vi "PIDController_AdvCalculate_FF_Sp_Pv_Per.vi"(6 "Period":dbl, 7 "Auto":bool=TRUE, 8 "FF":dbl, 9 "SP":dbl, 10 "PV":dbl, 11 "in PID_CONTROLLER":T1={"Kp"=0.0, "Ki"=0.0, "Kd"=0.0, "Period"=0.0, "Max_Integral"=0.0, "Min_Integral"=0.0, "Max_Input"=0.0, "Min_Input"=0.0, "Continuous"=FALSE, "PositionError"=0.0, "VelocityError"=0.0, "PrevError"=0.0, "TotalError"=0.0, "PositionTolerance"=0.0, "VelocityTolerance"=0.0, "SetPoint"=0.0, "Kf"=0.0, "Prev_Deriv"=0.0, "Prev_Deriv 2"=0.0, "DerivativeFilter"=FALSE, "Min_Output"=-9.99e+35, "Max_Output"=9.9e+35, "Prev_F_P"=0.0, "Prev_F_P_2"=0.0, "AntiWindupActive"=FALSE, "Measurement"=0.0} {"Measurement" format="%16_6e"; "Prev_F_P_2" format="%16_6e"; "Prev_F_P" format="%16_6e"; "Max_Output" format="%16_6e"; "Min_Output" format="%16_6e"; "Prev_Deriv 2" format="%16_6e"; "Prev_Deriv" format="%16_6e"; "Kf" format="%16_6e"; "SetPoint" format="%16_6e"; "VelocityTolerance" format="%16_6e"; "PositionTolerance" format="%16_6e"; "TotalError" format="%16_6e"; "PrevError" format="%16_6e"; "VelocityError" format="%16_6e"; "PositionError" format="%16_6e"; "Min_Input" format="%16_6e"; "Max_Input" format="%16_6e"; "Min_Integral" format="%16_6e"; "Max_Integral" format="%16_6e"; "Period" format="%16_6e"; "Kd" format="%16_6e"; "Ki" format="%16_6e"; "Kp" format="%16_6e"}) -> (1 "ControlOutput":dbl, 3 "out PID_CONTROLLER":T1={"Kp"=0.0, "Ki"=0.0, "Kd"=0.0, "Period"=0.0, "Max_Integral"=0.0, "Min_Integral"=0.0, "Max_Input"=0.0, "Min_Input"=0.0, "Continuous"=FALSE, "PositionError"=0.0, "VelocityError"=0.0, "PrevError"=0.0, "TotalError"=0.0, "PositionTolerance"=0.0, "VelocityTolerance"=0.0, "SetPoint"=0.0, "Kf"=0.0, "Prev_Deriv"=0.0, "Prev_Deriv 2"=0.0, "DerivativeFilter"=FALSE, "Min_Output"=-9.99e+35, "Max_Output"=9.9e+35, "Prev_F_P"=0.0, "Prev_F_P_2"=0.0, "AntiWindupActive"=FALSE, "Measurement"=0.0} {"Measurement" format="%16_6e"; "Prev_F_P_2" format="%16_6e"; "Prev_F_P" format="%16_6e"; "Max_Output" format="%16_6e"; "Min_Output" format="%16_6e"; "Prev_Deriv 2" format="%16_6e"; "Prev_Deriv" format="%16_6e"; "Kf" format="%16_6e"; "SetPoint" format="%16_6e"; "VelocityTolerance" format="%16_6e"; "PositionTolerance" format="%16_6e"; "TotalError" format="%16_6e"; "PrevError" format="%16_6e"; "VelocityError" format="%16_6e"; "PositionError" format="%16_6e"; "Min_Input" format="%16_6e"; "Max_Input" format="%16_6e"; "Min_Integral" format="%16_6e"; "Max_Integral" format="%16_6e"; "Period" format="%16_6e"; "Kd" format="%16_6e"; "Ki" format="%16_6e"; "Kp" format="%16_6e"})   [LabVIEW 2019, in "Trajectory_Library.lvlib"]
doc: "Returns the next output of the \"advanced\" PID controller. This controller implements the same PID as the \"normal\" controller with the following enhancements:\n - Integration by trapezoids is used.\n - Optionally filters derivative terms. (See SetDerivativeFilter subVI documentation for information.)\n - Incorporates optional feedforward.\n - Includes integral windup protection. This is only useful when output limits are specified.\n - When not called with a specific period, uses the actual elapsed time. (This subVI requires the call to pass the time period.) \n - Limits the outputs. When output limits are specified the output is cooerced be within these limits.\n - Includes an Auto/Manual mode. In manual mode the scaled feedforward is sent directly to the output and the PID controller tracks this output value to allow for smooth transition back to auto mode.\n\nThe generalized equation for this PID when in auto is:\n CO = Kf x feedforward + Kp x error + Ki x Integral(error) + Kd x Derivative(error)\n\nWhen auto mode is disabled, the generaized equation is:\n CO = Kf x feedforward \n \nInputs:\n - PID_Controller -- PID_Controller data cluster\n - PV-measurement -- The current measurement of the process variable. (PV)\n - SP-setpoint -- The new setpoint of the controller. (SP)\n - FF-feedforward -- Feedforward n the same units as the PV and SP\n - Period -- Period of this controller in seconds.\n - Auto -- Use the PID calculate when this is True\n\nOutputs:\n - PID_Controller -- Updated PID_Controller data cluster\n - CO-ControlOutput -- Controller output (CO)"
uses:
  Trajectory_Library.lvlib
  TypeDef/PID_CONTROLLER.ctl
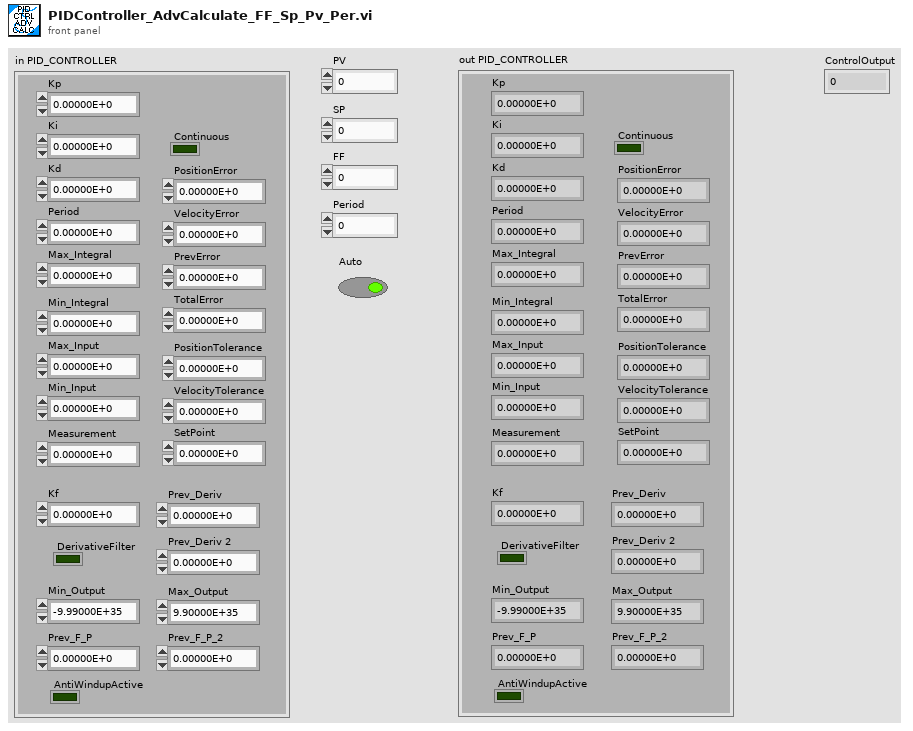
[diagram p1: front panel]
types:
  T1 = typedef "Trajectory_Library.lvlib/PID_CONTROLLER.ctl" = cluster{"Kp":dbl, "Ki":dbl, "Kd":dbl, "Period":dbl, "Max_Integral":dbl, "Min_Integral":dbl, "Max_Input":dbl, "Min_Input":dbl, "Continuous":bool, "PositionError":dbl, "VelocityError":dbl, "PrevError":dbl, "TotalError":dbl, "PositionTolerance":dbl, "VelocityTolerance":dbl, "SetPoint":dbl, "Kf":dbl, "Prev_Deriv":dbl, "Prev_Deriv 2":dbl, "DerivativeFilter":bool, "Min_Output":dbl, "Max_Output":dbl, "Prev_F_P":dbl, "Prev_F_P_2":dbl, "AntiWindupActive":bool, "Measurement":dbl}
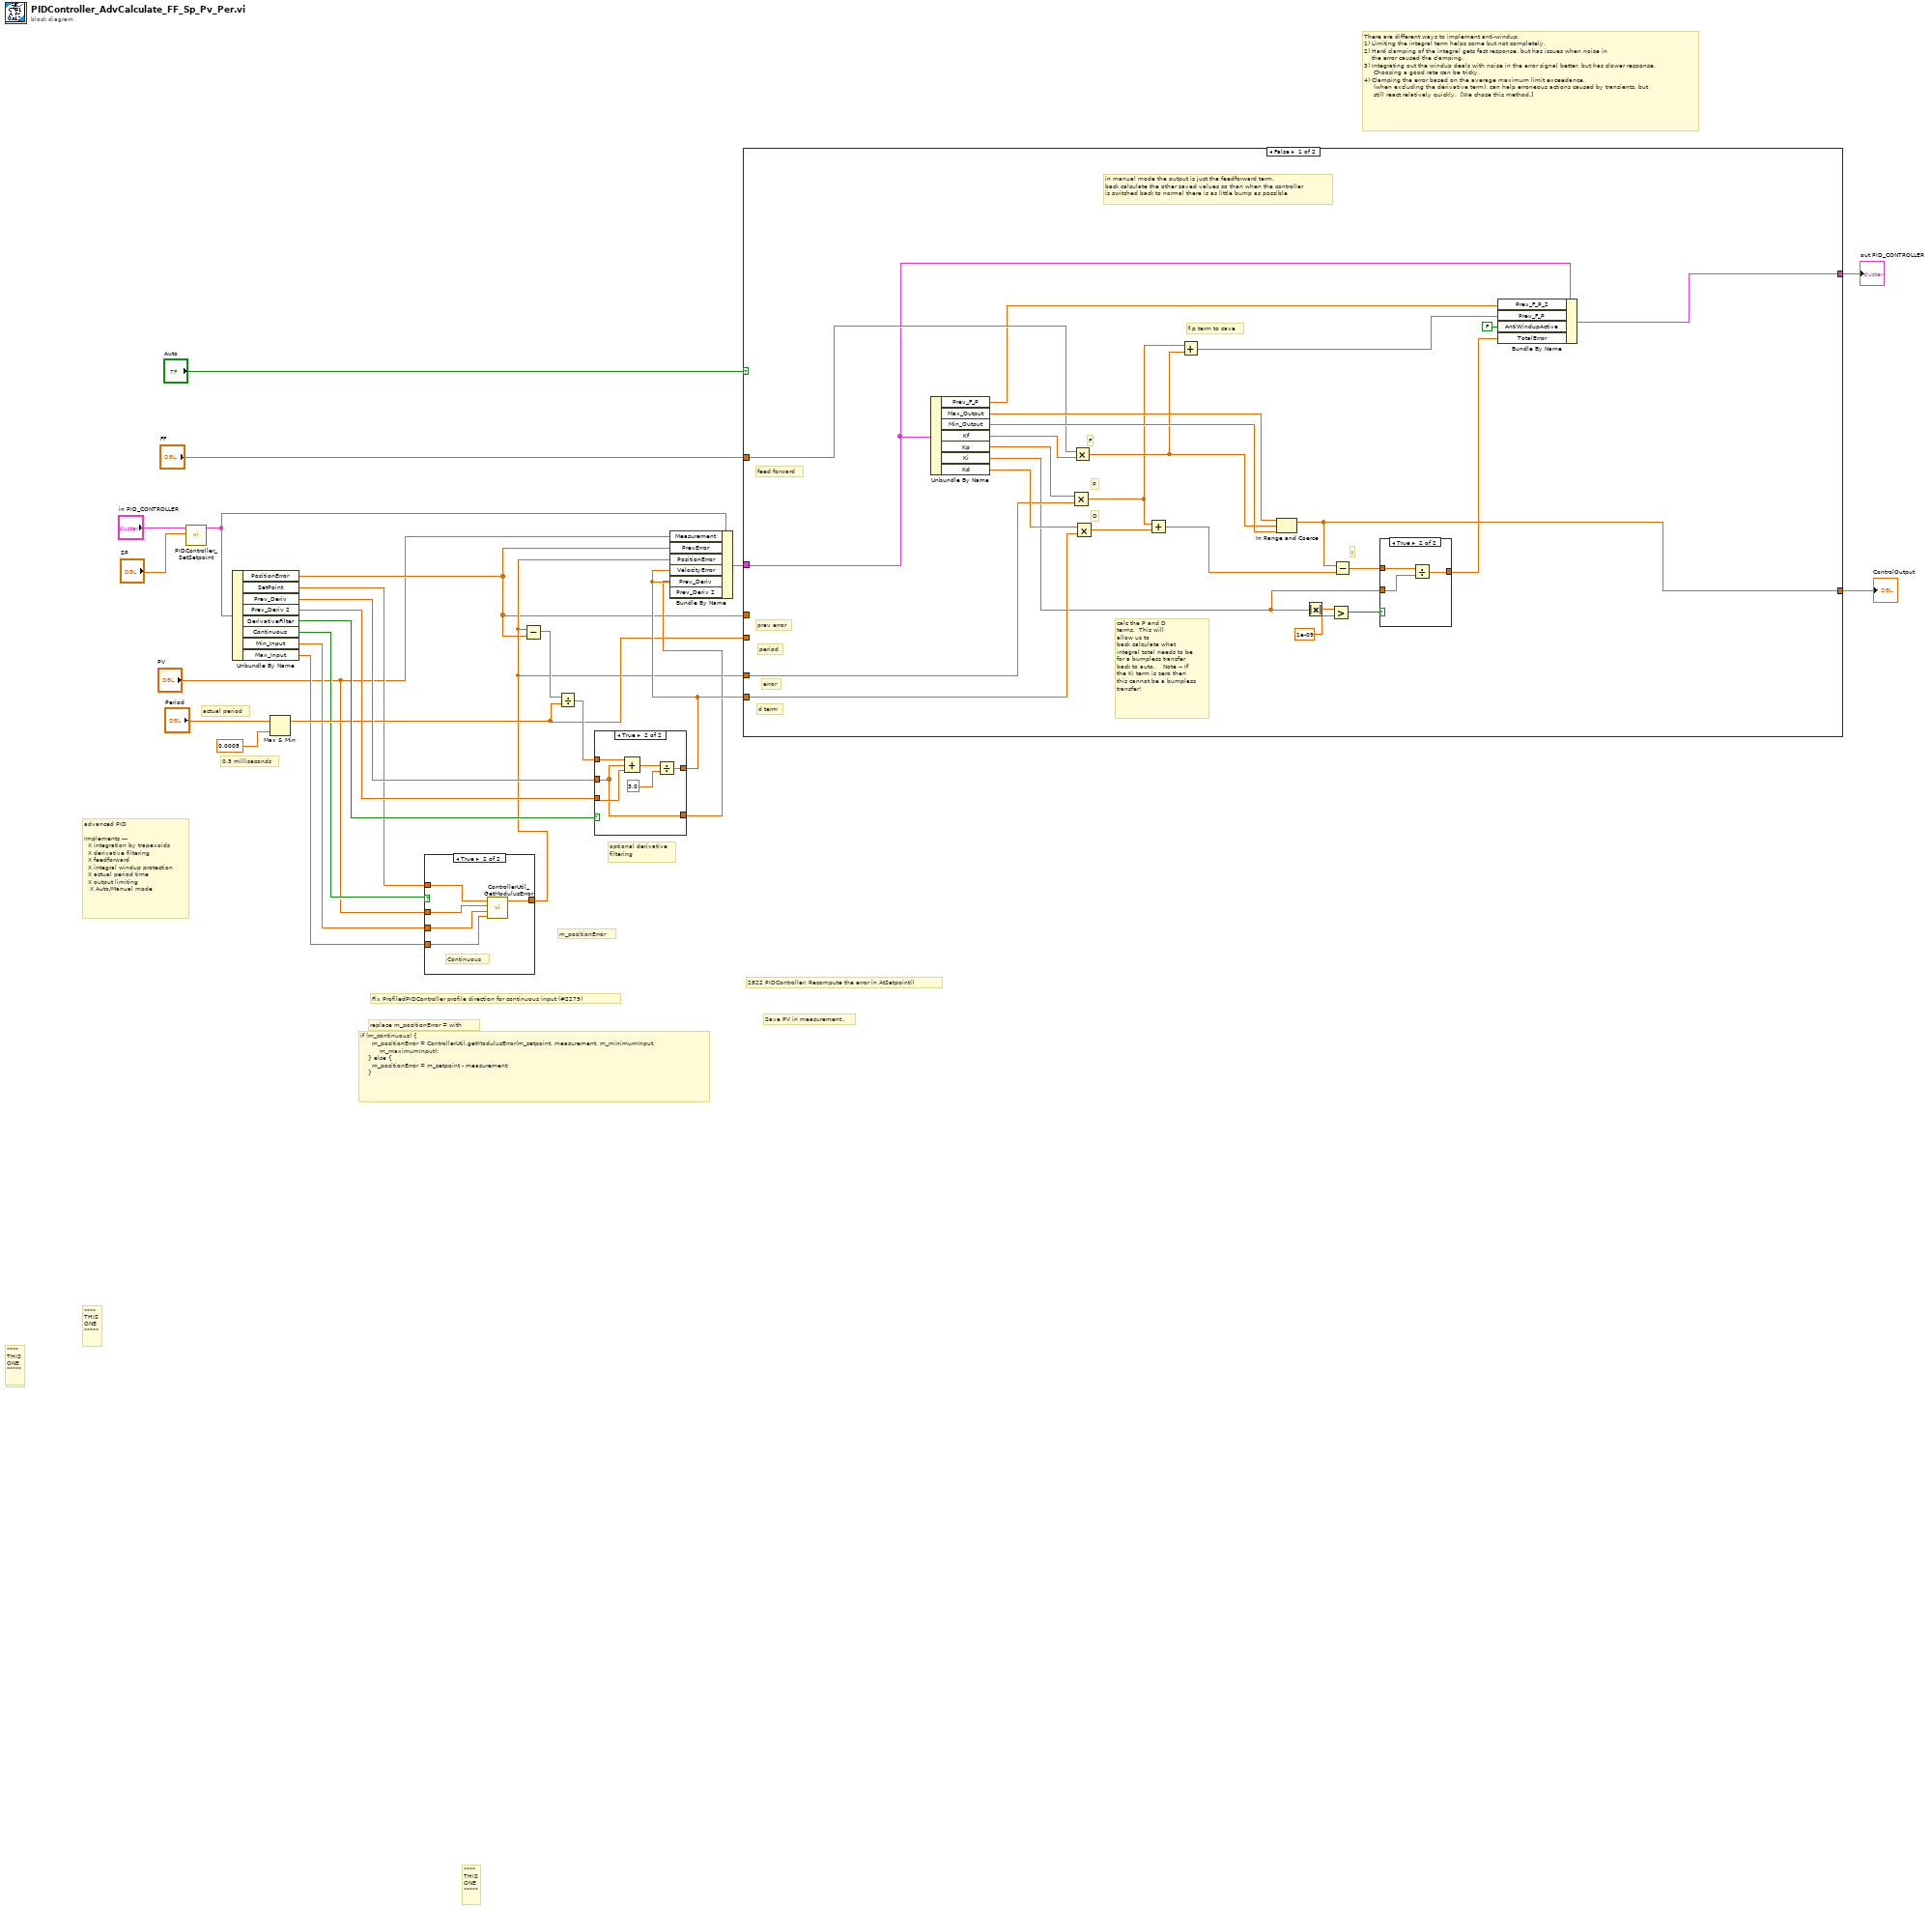
[diagram p0: block diagram]
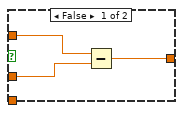
[diagram p2: hidden frame]
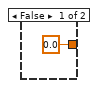
[diagram p3: hidden frame]
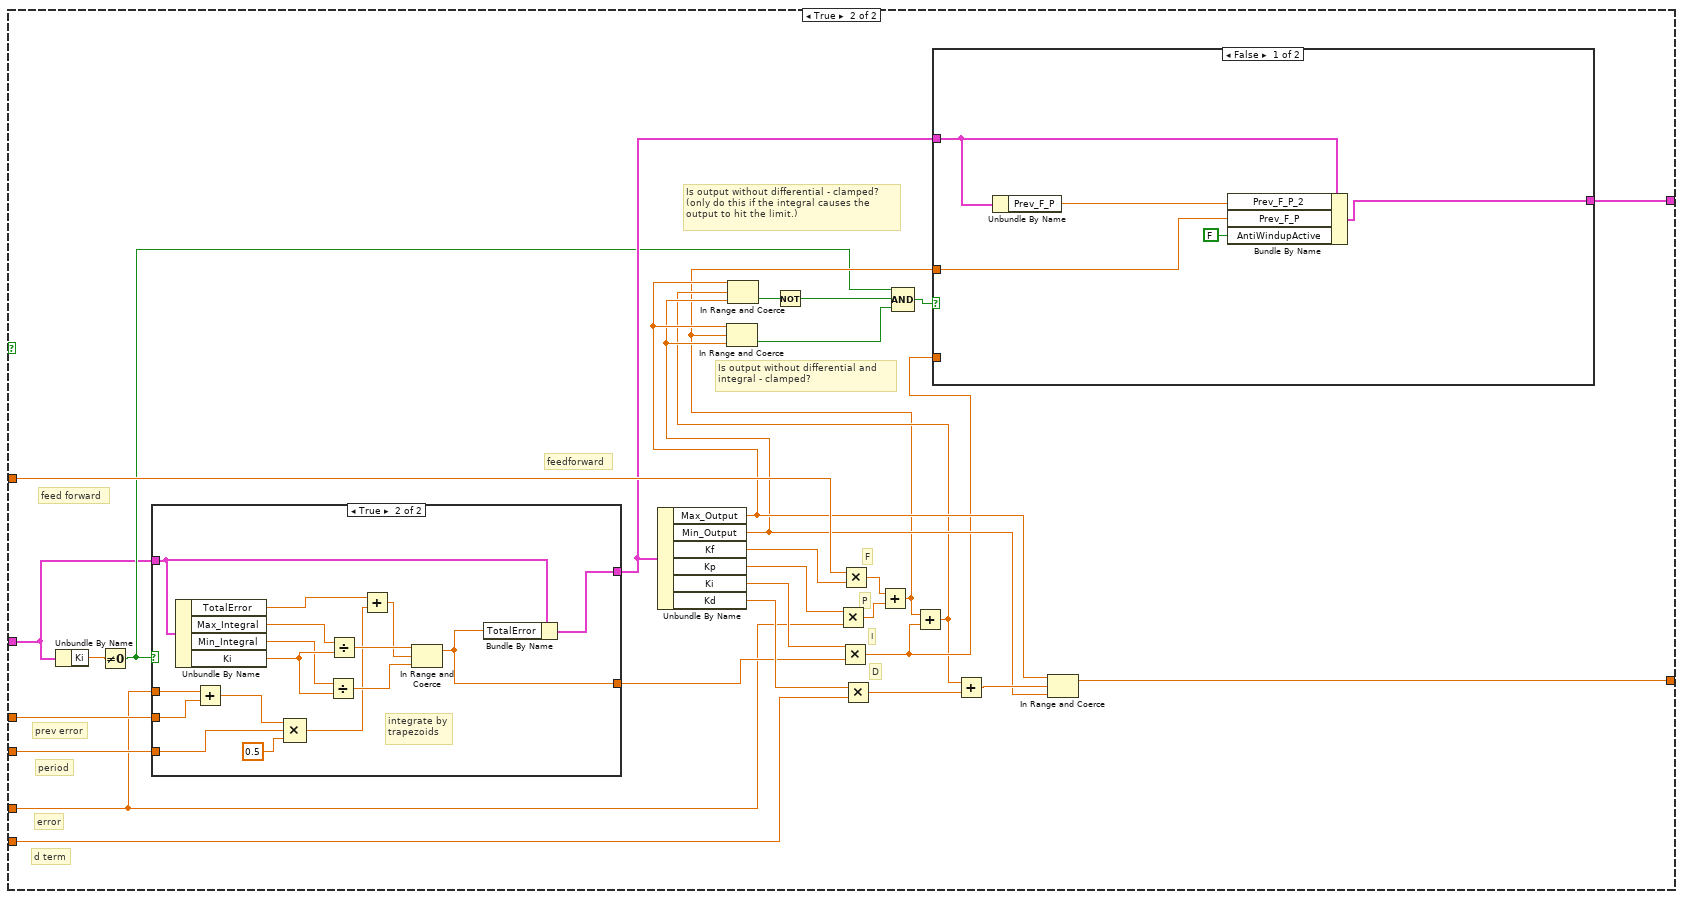
[diagram p4: hidden frame]
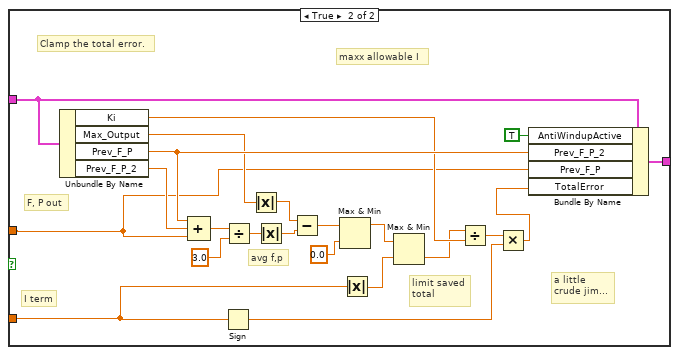
[diagram p5: hidden frame]
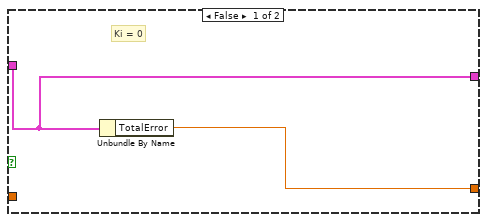
[diagram p6: hidden frame]
diagram:
  # "Save PV in measurement.."
  # "2822 PIDController: Recompute the error in AtSetpoint()"
  # "Fix ProfiledPIDController profile direction for continuous input (#2279)"
  # "replace m_positionError = with"
  # "if (m_continuous) {\n      m_positionError = ControllerUtil.getModulusError(m_setpoint, measurement, m_minimumInput,\n          m_maximumInput);\n    } else {\n      m_positionError = m_setpoint - measurement;\n    }"
  # "m_positionError"
  # "There are different ways to implement anti-windup. \n1) Limiting the integral term helps some but not completely.\n2) Hard clamping of the integral gets fast response, but has issues when noise in\n    the error caused the clamping.\n3) Integrating out the windup deals with noise in the error signal better, but has slower response.\n     Choosing a good rate can be tricky.\n4) Clamping the error based on the average maximum limit exceedance, \n     (when excluding the derivative term), can help erroneous actions caused by transients, but\n     still react relatively quickly.  [We chose this method.]"
  # "0.5 milliseconds"
  # "actual period"
  # "optional derivative\nfiltering"
  # "advanced PID\n\nImplements ---\n  X integration by trapexoids\n  X derivative filtering\n  X feedforward\n  X integral windup protection\n  X actual period time\n  X output limiting\n   X Auto/Manual mode"
  # "****\nTHIS\nONE\n*****"
  # "****\nTHIS\nONE\n*****"
  # "****\nTHIS\nONE\n*****"
  # "****\nTHIS\nONE\n*****"
  n1 = call "PIDController_SetSetpoint.vi"("Setpoint"="SP", "in PID_CONTROLLER"="in PID_CONTROLLER") -> ("out PID_CONTROLLER"=w1:T1)  [unwired: 9 in]
  n2 = Unbundle By Name(w1) -> ("PositionError"=w3:dbl, "SetPoint"=w8:dbl, "Prev_Deriv"=w18:dbl, "Prev_Deriv 2"=w19:dbl, "DerivativeFilter"=w21:bool, "Continuous"=w7:bool, "Min_Input"=w6:dbl, "Max_Input"=w5:dbl)
  n3 = Max & Min(x="Period", y=0.0005) -> (max(x,y)=w14:dbl)  [unwired: 1 out]
  n4 = case shown="True" w7 {
    tunnel: w8 -> [w28 w33]
    tunnel: "PV" -> [w27 w32]
    tunnel: [w26 w29] -> w4
    tunnel: w6 -> [_ w31]
    tunnel: w5 -> [_ w30]
    frame False {
      n5 = Subtract(x=w28, y=w27) -> (x-y=w26:dbl)
    }
    frame True {
      # "Continuous"
      n6 = call "ControllerUtil_GetModulusError.vi"("Maximum_Input"=w30, "Minimum_Input"=w31, "Measurerment(PV)"=w32, "Reference(SP)"=w33) -> ("Error"=w29:dbl)  [unwired: 7 in]
    }
  }
  n7 = Subtract(x=w4, y=w3) -> (x-y=w25:dbl)
  n8 = Divide(x=w25, y=w14) -> (x/y=w20:dbl)
  n9 = case shown="True" w21 {
    tunnel: w20 -> [w35 w41]
    tunnel: [w35 w38] -> w17
    tunnel: w19 -> [_ w40]
    tunnel: w18 -> [w34 w39]
    tunnel: [w34 w39] -> w16
    frame False {
    }
    frame True {
      n10 = Compound Arithmetic op=ADD(w41, w39, w40) -> (w36:dbl)
      n11 = Divide(x=w36, y=3.0) -> (x/y=w38:dbl)
    }
  }
  n12 = Bundle By Name(cluster=w1, "Measurement"="PV", "PrevError"=w3, "PositionError"=w4, "VelocityError"=w17, "Prev_Deriv"=w17, "Prev_Deriv 2"=w16) -> (w10:T1)
  n13 = case shown="False" "Auto" {
    tunnel: w3 -> [_ w93]
    tunnel: "FF" -> [w59 w92]
    tunnel: w17 -> [w58 w90]
    tunnel: w14 -> [_ w89]
    tunnel: [w56 w88] -> w12
    tunnel: [w48 w86] -> w11
    tunnel: w10 -> [w51 w71]
    tunnel: w4 -> [w57 w70]
    frame False {
      # "f,p term to save"
      # "I"
      # "calc the P and D\nterms.  This will \nallow us to \nback calculate what\nintegral total needs to be\nfor a bumpless transfer\nback to auto.    Note -- If\nthe Ki term is zero then \nthis cannot be a bumpless\ntransfer!"
      # "in manual mode the output is just the feedforward term.\nback calculate the other saved values so than when the controller\nis switched back to normal there is as little bump as possible"
      # "prev error"
      # "period"
      # "error"
      # "d term"
      # "feed forward"
      # "D"
      # "P"
      # "F"
      n14 = Unbundle By Name(w51) -> ("Prev_F_P"=w50:dbl, "Max_Output"=w61:dbl, "Min_Output"=w60:dbl, "Kf"=w63:dbl, "Kp"=w65:dbl, "Ki"=w43:dbl, "Kd"=w64:dbl)
      n15 = Multiply(x=w65, y=w57) -> (x*y=w53:dbl)
      n16 = Multiply(x=w59, y=w63) -> (x*y=w54:dbl)
      n17 = Multiply(x=w64, y=w58) -> (x*y=w62:dbl)
      n18 = Add(x=w53, y=w62) -> (x+y=w55:dbl)
      n19 = Add(x=w53, y=w54) -> (x+y=w49:dbl)
      n20 = In Range and Coerce(upper limit=w61, x=w54, lower limit=w60) -> (coerced(x)=w56:dbl)  [unwired: 1 out]
      n21 = Absolute Value(x=w43) -> (abs(x)=w47:dbl)
      n22 = Greater?(x=w47, y=1e-09) -> (0:w45:bool)
      n23 = Subtract(x=w56, y=w55) -> (x-y=w44:dbl)
      n24 = case shown="True" w45 {
        tunnel: w44 -> [_ w69]
        tunnel: w43 -> [_ w68]
        tunnel: [0.0 w67] -> w42
        frame False {
        }
        frame True {
          n25 = Divide(x=w69, y=w68) -> (x/y=w67:dbl)
        }
      }
      n26 = Bundle By Name(cluster=w51, "Prev_F_P_2"=w50, "Prev_F_P"=w49, "AntiWindupActive"=FALSE, "TotalError"=w42) -> (w48:T1)
    }
    frame True {
      # "feed forward"
      # "prev error"
      # "period"
      # "error"
      # "d term"
      # "D"
      # "I"
      # "P"
      # "F"
      # "Is output without differential and \nintegral - clamped?"
      # "Is output without differential - clamped?\n(only do this if the integral causes the \noutput to hit the limit.)"
      # "feedforward"
      n27 = Unbundle By Name(w71) -> ("Ki"=w98:dbl)
      n28 = Not Equal To 0?(x=w98) -> (x != 0?=w72:bool)
      n29 = case shown="True" w72 {
        tunnel: w71 -> [w126 w137]
        tunnel: [w126 w136] -> w87
        tunnel: [w127 w135] -> w94
        tunnel: w89 -> [_ w130]
        tunnel: w70 -> [_ w133]
        tunnel: w93 -> [_ w132]
        frame False {
          # "Ki = 0"
          n30 = Unbundle By Name(w126) -> ("TotalError"=w127:dbl)
        }
        frame True {
          # "integrate by\ntrapezoids"
          n31 = Unbundle By Name(w137) -> ("TotalError"=w134:dbl, "Max_Integral"=w142:dbl, "Min_Integral"=w141:dbl, "Ki"=w143:dbl)
          n32 = Add(x=w133, y=w132) -> (x+y=w131:dbl)
          n33 = Compound Arithmetic op=MULTIPLY(w131, w130, 0.5 ("value")) -> (w128:dbl)
          n34 = Divide(x=w141, y=w143) -> (x/y=w139:dbl)
          n35 = Divide(x=w142, y=w143) -> (x/y=w140:dbl)
          n36 = Add(x=w134, y=w128) -> (x+y=w138:dbl)
          n37 = In Range and Coerce(upper limit=w140, x=w138, lower limit=w139) -> (coerced(x)=w135:dbl)  [unwired: 1 out]
          n38 = Bundle By Name(cluster=w137, "TotalError"=w135) -> (w136:T1)
        }
      }
      n39 = Unbundle By Name(w87) -> ("Max_Output"=w81:dbl, "Min_Output"=w80:dbl, "Kf"=w91:dbl, "Kp"=w97:dbl, "Ki"=w96:dbl, "Kd"=w95:dbl)
      n40 = Multiply(x=w97, y=w70) -> (x*y=w82:dbl)
      n41 = Multiply(x=w96, y=w94) -> (x*y=w75:dbl)
      n42 = Multiply(x=w92, y=w91) -> (x*y=w83:dbl)
      n43 = Multiply(x=w95, y=w90) -> (x*y=w84:dbl)
      n44 = Add(x=w83, y=w82) -> (x+y=w73:dbl)
      n45 = In Range and Coerce(upper limit=w81, x=w73, lower limit=w80) -> (In Range?=w77:bool)  [unwired: 1 out]
      n46 = Add(x=w73, y=w75) -> (x+y=w74:dbl)
      n47 = In Range and Coerce(upper limit=w81, x=w74, lower limit=w80) -> (In Range?=w79:bool)  [unwired: 1 out]
      n48 = Not(x=w79) -> (.not. x?=w78:bool)
      n49 = Compound Arithmetic op=AND(w72, w78, w77) -> (w76:bool)
      n50 = case shown="False" w76 {
        tunnel: w87 -> [w103 w124]
        tunnel: [w101 w125] -> w86
        tunnel: w75 -> [_ w107]
        tunnel: w73 -> [w99 w110]
        frame False {
          n51 = Unbundle By Name(w103) -> ("Prev_F_P"=w102:dbl)
          n52 = Bundle By Name(cluster=w103, "Prev_F_P_2"=w102, "Prev_F_P"=w99, "AntiWindupActive"=FALSE) -> (w101:T1)
        }
        frame True {
          # "limit saved\ntotal"
          # "maxx allowable I"
          # "a little\ncrude jim..."
          # "avg f,p"
          # "F, P out"
          # "I term"
          # "Clamp the total error."
          n53 = Unbundle By Name(w124) -> ("Ki"=w115:dbl, "Max_Output"=w119:dbl, "Prev_F_P"=w120:dbl, "Prev_F_P_2"=w118:dbl)
          n54 = Compound Arithmetic op=ADD(w120, w118, w110) -> (w123:dbl)
          n55 = Sign(1:w107) -> (0:w112:dbl)
          n56 = Divide(x=w123, y=3.0) -> (x/y=w121:dbl)
          n57 = Absolute Value(x=w119) -> (abs(x)=w108:dbl)
          n58 = Absolute Value(x=w121) -> (abs(x)=w109:dbl)
          n59 = Subtract(x=w108, y=w109) -> (x-y=w117:dbl)
          n60 = Max & Min(x=w117, y=0.0) -> (max(x,y)=w106:dbl)  [unwired: 1 out]
          n61 = Absolute Value(x=w107) -> (abs(x)=w105:dbl)
          n62 = Max & Min(x=w106, y=w105) -> (min(x,y)=w104:dbl)  [unwired: 1 out]
          n63 = Divide(x=w104, y=w115) -> (x/y=w114:dbl)
          n64 = Multiply(x=w114, y=w112) -> (x*y=w113:dbl)
          n65 = Bundle By Name(cluster=w124, "AntiWindupActive"=TRUE, "Prev_F_P_2"=w120, "Prev_F_P"=w110, "TotalError"=w113) -> (w125:T1)
        }
      }
      n66 = Add(x=w74, y=w84) -> (x+y=w85:dbl)
      n67 = In Range and Coerce(upper limit=w81, x=w85, lower limit=w80) -> (coerced(x)=w88:dbl)  [unwired: 1 out]
    }
  }
  "out PID_CONTROLLER" <- w11
  "ControlOutput" <- w12
